vi "Sort Project Items.vi"(6 "Slide in":refnum<vi>, 10 "Project Items":refnum<vi>[](array[refnum]), 11 "Sorted VIs in":T1) -> (3 "Sorted VIs out":T1)   [LabVIEW 2014]
uses:
  Type Defs/TYPE_Sorted Project Items.ctl
  Type Defs/TYPE_Sorter States.ctl
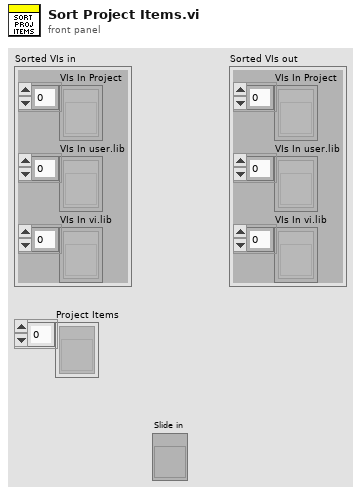
[diagram p1: front panel]
types:
  T1 = typedef "TYPE_Sorted Project Items.ctl" = cluster{"VIs In Project":refnum<vi>[], "VIs In user.lib":refnum<vi>[], "VIs In vi.lib":refnum<vi>[]}
  T2 = typedef "TYPE_Sorter States.ctl" = enum16{"Filter VIs", "Check VI Lib", "Check User Lib", "Add Project Lib", "Finish"}
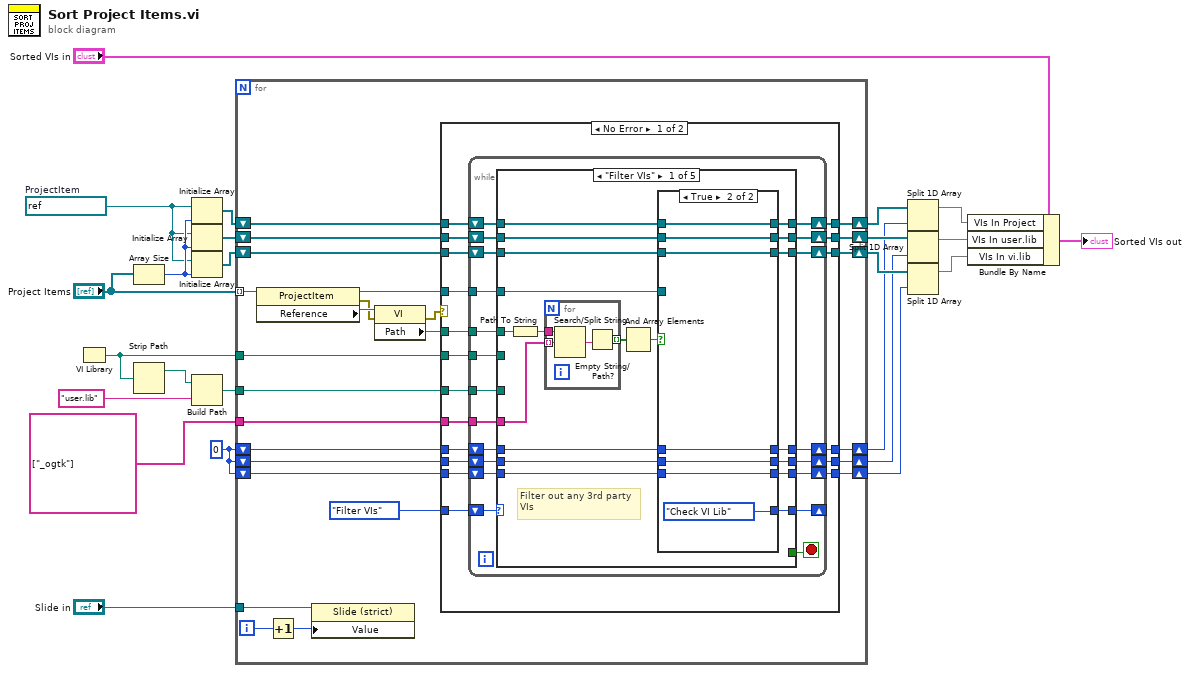
[diagram p0: block diagram]
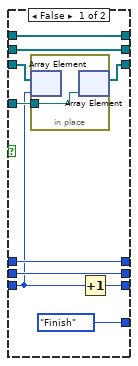
[diagram p2: hidden frame]
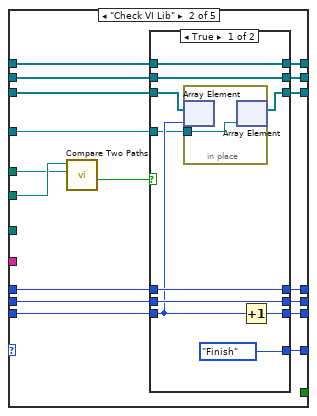
[diagram p3: hidden frame]
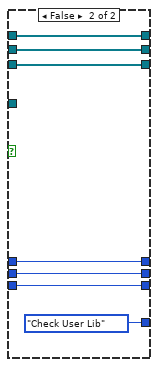
[diagram p4: hidden frame]
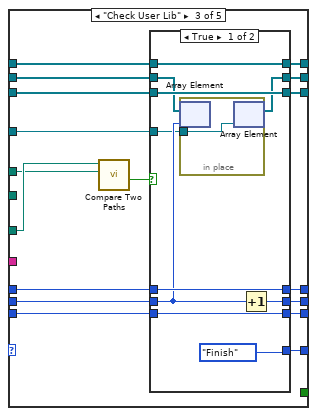
[diagram p5: hidden frame]
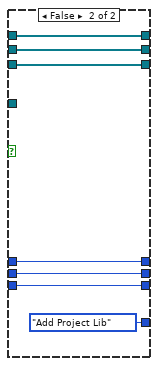
[diagram p6: hidden frame]
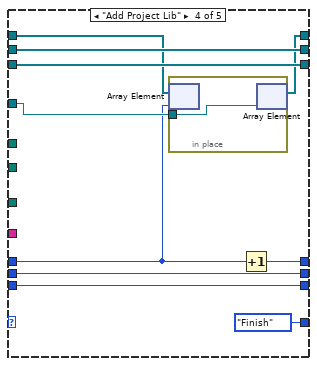
[diagram p7: hidden frame]
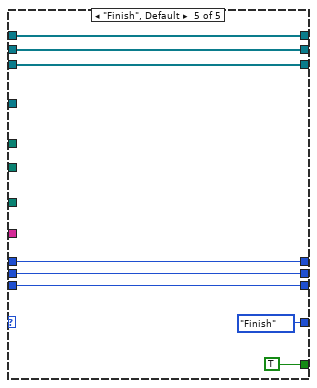
[diagram p8: hidden frame]
diagram:
  w12 = 0
  w13 = refnum<vi> refnum  # ProjectItem
  n1 = VI Library() -> (path=w20:path)
  n2 = Array Size(array="Project Items") -> (size(s)=w14:i32)
  n3 = Strip Path(path=w20) -> (stripped path=w22:path)  [unwired: 1 out]
  n4 = Initialize Array(w13, w14) -> (w18:refnum<vi>[])
  n5 = Initialize Array(w13, w14) -> (w17:refnum<vi>[])
  n6 = Initialize Array(w13, w14) -> (w16:refnum<vi>[])
  n7 = Build Path(base path=w22, name or relative path="user.lib") -> (appended path=w19:path)
  n8 = for {
    shift-right: [w47] -> w8
    shift-left: w18 -> [w48]
    shift-right: [w44] -> w7
    shift-left: w17 -> [w46]
    shift-right: [w43] -> w6
    shift-left: w16 -> [w45]
    tunnel: "Project Items" -> [w49] mode=indexing
    tunnel: w20 -> [w39]
    tunnel: w19 -> [w38]
    shift-right: [w37] -> w3
    shift-left: w12 -> [w36]
    shift-right: [w35] -> w5
    shift-left: w12 -> [w34]
    shift-right: [w33] -> w4
    shift-left: w12 -> [w32]
    tunnel: string[] ["_ogtk"] -> [w30]
    tunnel: "Slide in" -> [w29]
    i -> [w28]
    n9 = property class="ProjectItem"(reference=w49) -> (reference out=w40:refnum<vi>, error out=w25:errorcluster, "Reference"=w42:refnum<vi>)  [unwired: 1 in]
    n10 = Increment(x=w28) -> (x+1=w27:i32)
    n11 = property on="Property Node" class="Slide (strict)"(reference=w29, "Value"=w27) -> ()  [unwired: 1 in, 2 out]
    n12 = property class="VI"(reference=w42, error in=w25) -> (error out=w26:errorcluster, "Path"=w31:path)  [unwired: 1 out]
    n13 = case shown="No Error" w26 {
      tunnel: w48 -> [w67 w223]
      tunnel: [w66 w223] -> w47
      tunnel: w46 -> [w65 w222]
      tunnel: w45 -> [w64 w221]
      tunnel: [w63 w222] -> w44
      tunnel: [w62 w221] -> w43
      tunnel: TYPE_Sorter_States."Filter VIs" -> [w61 _]
      tunnel: w40 -> [w60 _]
      tunnel: w39 -> [w59 _]
      tunnel: w38 -> [w58 _]
      tunnel: [w57 w220] -> w37
      tunnel: w36 -> [w56 w220]
      tunnel: [w55 w219] -> w35
      tunnel: w34 -> [w54 w219]
      tunnel: [w53 w218] -> w33
      tunnel: w32 -> [w52 w218]
      tunnel: w31 -> [w51 _]
      tunnel: w30 -> [w50 _]
      frame No Error {
        n14 = while {
          shift-right: [w80] -> w66
          shift-left: w67 -> [w83]
          shift-right: [w79] -> w63
          shift-left: w65 -> [w82]
          shift-right: [w78] -> w62
          shift-left: w64 -> [w81]
          tunnel: w51 -> [w87]
          shift-right: [w85] -> _
          shift-left: w61 -> [w86]
          tunnel: w60 -> [w77]
          tunnel: w59 -> [w76]
          tunnel: w58 -> [w75]
          shift-right: [w74] -> w57
          shift-left: w56 -> [w73]
          shift-right: [w72] -> w55
          shift-left: w54 -> [w71]
          shift-right: [w70] -> w53
          shift-left: w52 -> [w69]
          tunnel: w50 -> [w68]
          stop <- w84 stop-if-true
          n15 = case shown="\"Filter VIs\"" w86 {
            tunnel: w87 -> [w92 w129 w164 _ _]
            tunnel: [w99 w138 w173 TYPE_Sorter_States."Finish" TYPE_Sorter_States."Finish"] -> w85
            tunnel: [_ _ _ _ TRUE] -> w84
            tunnel: w83 -> [w100 w139 w174 w202 w216]
            tunnel: w82 -> [w102 w141 w176 w208 w215]
            tunnel: w81 -> [w105 w144 w179 w207 w214]
            tunnel: [w101 w140 w175 w201 w216] -> w80
            tunnel: [w103 w142 w177 w208 w215] -> w79
            tunnel: [w106 w145 w180 w207 w214] -> w78
            tunnel: w77 -> [w104 w143 w178 w200 _]
            tunnel: w76 -> [_ w130 _ _ _]
            tunnel: w75 -> [_ _ w165 _ _]
            tunnel: [w98 w137 w172 w206 w213] -> w74
            tunnel: w73 -> [w97 w136 w171 w199 w213]
            tunnel: [w96 w135 w170 w205 w212] -> w72
            tunnel: w71 -> [w95 w134 w169 w205 w212]
            tunnel: [w94 w133 w168 w204 w211] -> w70
            tunnel: w69 -> [w93 w132 w167 w204 w211]
            tunnel: w68 -> [w90 _ _ _ _]
            frame "Filter VIs" {
              # "Filter out any 3rd party\nVIs"
              n16 = Path To String(path=w92) -> (string=w91:string)
              n17 = for {
                tunnel: w91 -> [w110]
                tunnel: w90 -> [w109] mode=indexing
                tunnel: [w107] -> w89 mode=indexing
                n18 = Search/Split String(string=w110, search string/char (-)=w109) -> (match + rest of string=w108:string)  [unwired: 1 in, 2 out]
                n19 = Empty String/Path?(string/path=w108) -> (empty?=w107:bool)
              }
              n20 = And Array Elements(Boolean array=w89) -> (logical AND=w88:bool)
              n21 = case shown="True" w88 {
                tunnel: [w112 w126] -> w106
                tunnel: w105 -> [w113 w126]
                tunnel: w104 -> [w118 _]
                tunnel: [w120 w127] -> w103
                tunnel: w102 -> [w120 w127]
                tunnel: [w119 w128] -> w101
                tunnel: w100 -> [w119 w128]
                tunnel: [TYPE_Sorter_States."Finish" TYPE_Sorter_States."Check VI Lib"] -> w99
                tunnel: [w114 w125] -> w98
                tunnel: w97 -> [w114 w125]
                tunnel: [w117 w124] -> w96
                tunnel: w95 -> [w117 w124]
                tunnel: [w116 w123] -> w94
                tunnel: w93 -> [w111 w123]
                frame False {
                  n22 = in-place {
                    in-place-border: w118 -> [w121]
                    n23 = in-place-array #1(w113, w111) -> ()  [unwired: 1 out]
                    n24 = in-place-array #1(w121) -> (w112:refnum<vi>[])  [unwired: 1 out]
                  }
                  n25 = Increment(x=w111) -> (x+1=w116:i32)
                }
                frame True {
                }
              }
            }
            frame "Check VI Lib" {
              n26 = call <vilib>:"Compare Two Paths.vi"("Path 2"=w129, "Path 1"=w130) -> ("Path 2 Relative to Path 1?"=w131:bool)  [unwired: 6 in, 3 out]
              n27 = case shown="True" w131 {
                tunnel: [w147 w161] -> w145
                tunnel: w144 -> [w149 w161]
                tunnel: w143 -> [w146 _]
                tunnel: [w155 w162] -> w142
                tunnel: w141 -> [w155 w162]
                tunnel: [w154 w163] -> w140
                tunnel: w139 -> [w154 w163]
                tunnel: [TYPE_Sorter_States."Finish" TYPE_Sorter_States."Check User Lib"] -> w138
                tunnel: [w153 w160] -> w137
                tunnel: w136 -> [w153 w160]
                tunnel: [w152 w159] -> w135
                tunnel: w134 -> [w152 w159]
                tunnel: [w151 w158] -> w133
                tunnel: w132 -> [w148 w158]
                frame True {
                  n28 = in-place {
                    in-place-border: w146 -> [w156]
                    n29 = in-place-array #2(w149, w148) -> ()  [unwired: 1 out]
                    n30 = in-place-array #2(w156) -> (w147:refnum<vi>[])  [unwired: 1 out]
                  }
                  n31 = Increment(x=w148) -> (x+1=w151:i32)
                }
                frame False {
                }
              }
            }
            frame "Check User Lib" {
              n32 = call <vilib>:"Compare Two Paths.vi"("Path 2"=w164, "Path 1"=w165) -> ("Path 2 Relative to Path 1?"=w166:bool)  [unwired: 6 in, 3 out]
              n33 = case shown="True" w166 {
                tunnel: [w189 w196] -> w180
                tunnel: w179 -> [w189 w196]
                tunnel: w178 -> [w181 _]
                tunnel: [w183 w197] -> w177
                tunnel: w176 -> [w184 w197]
                tunnel: [w190 w198] -> w175
                tunnel: w174 -> [w190 w198]
                tunnel: [TYPE_Sorter_States."Finish" TYPE_Sorter_States."Add Project Lib"] -> w173
                tunnel: [w188 w195] -> w172
                tunnel: w171 -> [w188 w195]
                tunnel: [w186 w194] -> w170
                tunnel: w169 -> [w182 w194]
                tunnel: [w187 w193] -> w168
                tunnel: w167 -> [w187 w193]
                frame True {
                  n34 = in-place {
                    in-place-border: w181 -> [w191]
                    n35 = in-place-array #3(w184, w182) -> ()  [unwired: 1 out]
                    n36 = in-place-array #3(w191) -> (w183:refnum<vi>[])  [unwired: 1 out]
                  }
                  n37 = Increment(x=w182) -> (x+1=w186:i32)
                }
                frame False {
                }
              }
            }
            frame "Add Project Lib" {
              n38 = in-place {
                in-place-border: w200 -> [w209]
                n39 = in-place-array #4(w202, w199) -> ()  [unwired: 1 out]
                n40 = in-place-array #4(w209) -> (w201:refnum<vi>[])  [unwired: 1 out]
              }
              n41 = Increment(x=w199) -> (x+1=w206:i32)
            }
            frame "Finish", Default {
            }
          }
        }
      }
      frame Error {
      }
    }
  }
  n42 = Split 1D Array(array=w8, index=w3) -> (first subarray=w11:refnum<vi>[])  [unwired: 1 out]
  n43 = Split 1D Array(array=w7, index=w5) -> (first subarray=w10:refnum<vi>[])  [unwired: 1 out]
  n44 = Split 1D Array(array=w6, index=w4) -> (first subarray=w9:refnum<vi>[])  [unwired: 1 out]
  n45 = Bundle By Name(cluster="Sorted VIs in", "VIs In Project"=w11, "VIs In user.lib"=w10, "VIs In vi.lib"=w9) -> (→"Sorted VIs out":T1)
